vi "tsc-error-example-main.vi"() -> ()   [LabVIEW 2019]
uses:
  TSC Error.lvlib
panel:
  in  "Stop":bool
  out "header":bool
  in  "error":bool
  # "Run VI -> press button to see the error propagated to the message handling loop"
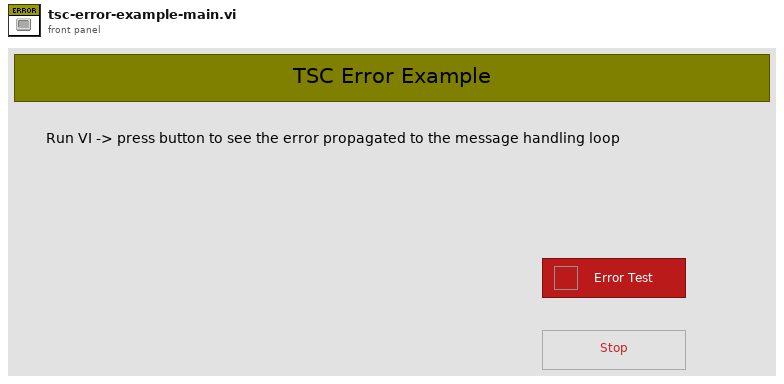
[diagram p1: front panel]
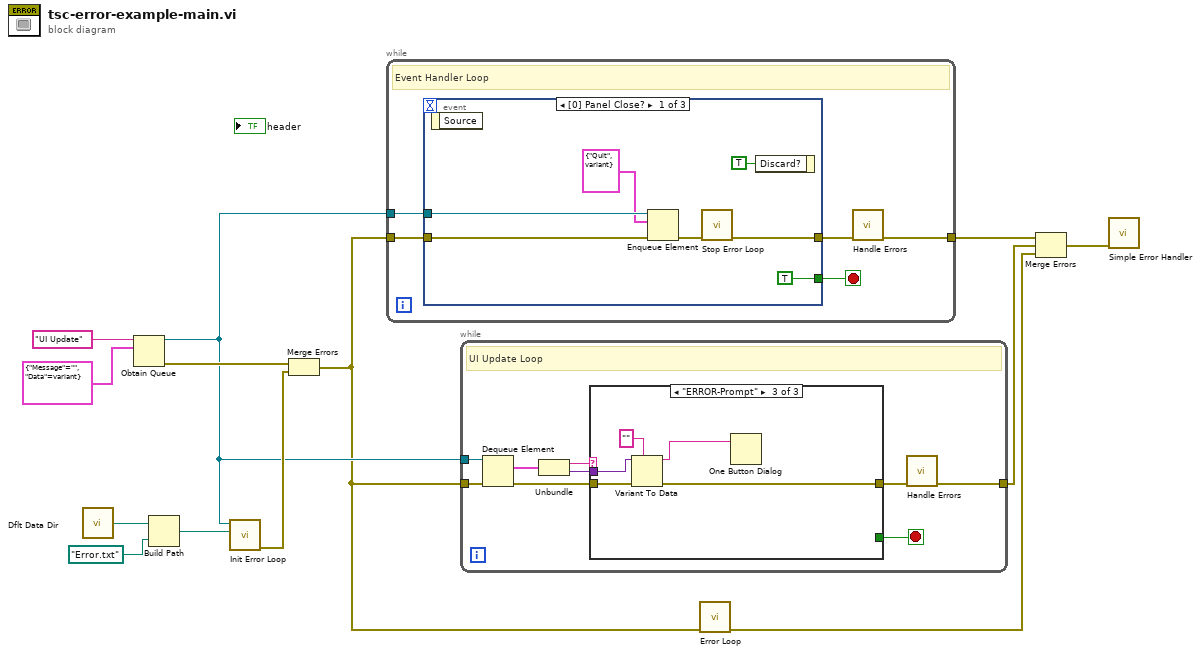
[diagram p0: block diagram]
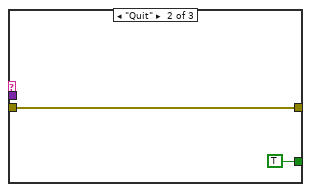
[diagram p3: hidden frame]
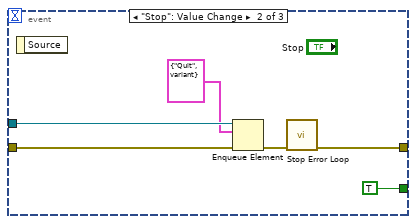
[diagram p4: hidden frame]
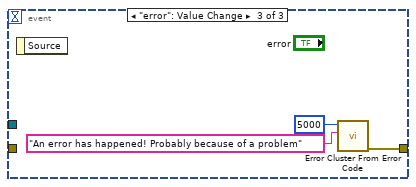
[diagram p5: hidden frame]
diagram:
  n1 = call <vilib>:"Dflt Data Dir.vi"() -> ("App:Default Data Directory"=w1:path)
  n2 = Obtain Queue(name (unnamed)="UI Update", element data type=cluster{"Message":string, "Data":variant} {"Message"="", "Data"=variant}) -> (queue out=w9:refnum<queue>, error out=w11:errorcluster)  [unwired: 3 in, 1 out]
  n3 = Build Path(base path=w1, name or relative path=path "Error.txt") -> (appended path=w2:path)
  n4 = call "Init Error Loop.vi"("Error Log"=w2, "Update Queue"=w9) -> ("Error Out"=w10:errorcluster)  [unwired: 9 in]
  n5 = Merge Errors(w11, w10) -> (w8:errorcluster)
  n6 = while {
    tunnel: w8 -> [w17]
    tunnel: [w15] -> w6
    tunnel: w9 -> [w14]
    stop <- w18 stop-if-true
    # "Event Handler Loop"
    n7 = event shown="[0] Panel Close?" {
      selector: _ -> [_ _ _]
      dyn-events: _ -> [_ _ _]
      timeout: _ -> [_ _ _]
      tunnel: [TRUE TRUE _] -> w18
      tunnel: w17 -> [w23 w30 _]
      tunnel: [w19 w26 w34] -> w16
      tunnel: w14 -> [w22 w29 _]
      event Panel Close? {
        n8 = event-data() -> ()  [unwired: 1 in, 1 out]
        n9 = Enqueue Element(queue=w22, element=cluster{"Message":string, "Data":variant} {"Message"="Quit", "Data"=variant}, error in (no error)=w23) -> (error out=w20:errorcluster)  [unwired: 1 in, 2 out]
        n10 = call "Stop Error Loop.vi"("Error In"=w20) -> ("Error Out"=w19:errorcluster)  [unwired: 10 in]
        n11 = event-data("Discard?"=TRUE) -> ()  [unwired: 1 in, 1 out]
      }
      event "Stop": Value Change {
        n12 = event-data() -> ()  [unwired: 1 in, 1 out]
        n13 = Enqueue Element(queue=w29, element=cluster{"Message":string, "Data":variant} {"Message"="Quit", "Data"=variant}, error in (no error)=w30) -> (error out=w27:errorcluster)  [unwired: 1 in, 2 out]
        n14 = call "Stop Error Loop.vi"("Error In"=w27) -> ("Error Out"=w26:errorcluster)  [unwired: 10 in]
      }
      event "error": Value Change {
        n15 = event-data() -> ()  [unwired: 1 in, 1 out]
        n16 = call <vilib>:"Error Cluster From Error Code.vi"("error message (\"\")"="An error has happened! Probably because of a problem" ("error message (\"\")"), "error code (0)"=5000) -> ("error out"=w34:errorcluster)  [unwired: 7 in]
      }
    }
    n17 = call "Handle Errors.vi"("error in (no error)"=w16) -> ("error out"=w15:errorcluster)  [unwired: 10 in]
  }
  n18 = while {
    tunnel: w9 -> [w43]
    tunnel: w8 -> [w42]
    tunnel: [w35] -> w7
    stop <- w37 stop-if-true
    # "UI Update Loop"
    n19 = Dequeue Element(queue=w43, error in (no error)=w42) -> (element=w40:cluster{"Message":string, "Data":variant}, error out=w41:errorcluster)  [unwired: 1 in, 2 out]
    n20 = Unbundle(w40) -> ("Message"=w39:string, "Data"=w38:variant)
    n21 = case shown="\"ERROR-Prompt\"" w39 {
      tunnel: w41 -> [w44 w45 w51]
      tunnel: w38 -> [_ _ w49]
      tunnel: [_ TRUE _] -> w37
      tunnel: [w44 w45 w50] -> w36
      frame Default {
      }
      frame "Quit" {
      }
      frame "ERROR-Prompt" {
        n22 = Variant To Data(error in=w51, type="", Variant=w49) -> (data=w47:string, error out=w50:errorcluster)
        n23 = One Button Dialog(message=w47) -> ()  [unwired: 1 in, 1 out]
      }
    }
    n24 = call "Handle Errors.vi"("error in (no error)"=w36) -> ("error out"=w35:errorcluster)  [unwired: 10 in]
  }
  n25 = call "Error Loop.vi"("error in"=w8) -> ("error out"=w5:errorcluster)  [unwired: 10 in]
  n26 = Merge Errors(w6, w7, w5) -> (w4:errorcluster)
  n27 = call <vilib>:"Simple Error Handler.vi"("error in (no error)"=w4) -> ()  [unwired: 4 in, 5 out]
